vi "driveCode.vi"(6 "tankJoystick":enum16{"xbox", "twoJoystick"}(ring), 7 "mode":enum16{"Tank", "Split Arcade", "Arcade"}(ring)=enum."Arcade", 8 "driverJoystick2":T1={"Device"=enum."USB 1"}, 9 "driverJoystick1":T1={"Device"=enum."USB 1"}, 10 "rightDrive":T3={"DeviceStatus"={"status"=FALSE, "code"=0, "source"=""}, "Type"=enum."PWM", "PWM"={"PWM Channel"=enum."Invalid", "DeadBand"={"Name"="", "maxPositivePwm"=0, "minPositivePwm"=0, "centerPwm"=0, "maxNegativePwm"=0, "minNegativePwm"=0, "angularRange"=0}}, "CAN"={"Device Number"=0, "SetOutput VI Ref"=variant(refnum<vi> refnum), "GetOutput VI Ref"=variant(refnum<vi> refnum), "Enable VI Ref"=variant(refnum<vi> refnum), "Disable VI Ref"=variant(refnum<vi> refnum), "Data"=variant}, "Invert"=FALSE, "DIO PWM"={"PWM \"Enable\" Channel"=enum."Invalid", "DIOChannel"=enum."Invalid", "PWM Rate"=0.0}}, 11 "leftDrive":T3={"DeviceStatus"={"status"=FALSE, "code"=0, "source"=""}, "Type"=enum."PWM", "PWM"={"PWM Channel"=enum."Invalid", "DeadBand"={"Name"="", "maxPositivePwm"=0, "minPositivePwm"=0, "centerPwm"=0, "maxNegativePwm"=0, "minNegativePwm"=0, "angularRange"=0}}, "CAN"={"Device Number"=0, "SetOutput VI Ref"=variant(refnum<vi> refnum), "GetOutput VI Ref"=variant(refnum<vi> refnum), "Enable VI Ref"=variant(refnum<vi> refnum), "Disable VI Ref"=variant(refnum<vi> refnum), "Data"=variant}, "Invert"=FALSE, "DIO PWM"={"PWM \"Enable\" Channel"=enum."Invalid", "DIOChannel"=enum."Invalid", "PWM Rate"=0.0}}) -> (0 "rightSpeed (%)":dbl, 1 "rightDrive":T3={"DeviceStatus"={"status"=FALSE, "code"=0, "source"=""}, "Type"=enum."PWM", "PWM"={"PWM Channel"=enum."Invalid", "DeadBand"={"Name"="", "maxPositivePwm"=0, "minPositivePwm"=0, "centerPwm"=0, "maxNegativePwm"=0, "minNegativePwm"=0, "angularRange"=0}}, "CAN"={"Device Number"=0, "SetOutput VI Ref"=variant(refnum<vi> refnum), "GetOutput VI Ref"=variant(refnum<vi> refnum), "Enable VI Ref"=variant(refnum<vi> refnum), "Disable VI Ref"=variant(refnum<vi> refnum), "Data"=variant}, "Invert"=FALSE, "DIO PWM"={"PWM \"Enable\" Channel"=enum."Invalid", "DIOChannel"=enum."Invalid", "PWM Rate"=0.0}}, 2 "leftSpeed (%)":dbl, 3 "leftDrive":T3={"DeviceStatus"={"status"=FALSE, "code"=0, "source"=""}, "Type"=enum."PWM", "PWM"={"PWM Channel"=enum."Invalid", "DeadBand"={"Name"="", "maxPositivePwm"=0, "minPositivePwm"=0, "centerPwm"=0, "maxNegativePwm"=0, "minNegativePwm"=0, "angularRange"=0}}, "CAN"={"Device Number"=0, "SetOutput VI Ref"=variant(refnum<vi> refnum), "GetOutput VI Ref"=variant(refnum<vi> refnum), "Enable VI Ref"=variant(refnum<vi> refnum), "Disable VI Ref"=variant(refnum<vi> refnum), "Data"=variant}, "Invert"=FALSE, "DIO PWM"={"PWM \"Enable\" Channel"=enum."Invalid", "DIOChannel"=enum."Invalid", "PWM Rate"=0.0}})   [LabVIEW 2017]
uses:
  <vilib>/Rock Robotics/WPI/MotorControl/WPI_MotorControlDeviceRef.ctl
  <vilib>/Rock Robotics/WPI/MotorControl/WPI_MotorControlType.ctl
  <vilib>/Rock Robotics/SystemInterfaces/DIO/FPGA_DIOPWMChannel.ctl
  <vilib>/Rock Robotics/WPI/PWM/WPI_PWMDeadband.ctl
  <vilib>/Rock Robotics/SystemInterfaces/DIO/FPGA_DIOChannel.ctl
  <vilib>/Rock Robotics/WPI/Joystick/WPI_JoystickDevRef.ctl
  <vilib>/Rock Robotics/WPI/Joystick/WPI_JoystickDeviceEnum.ctl
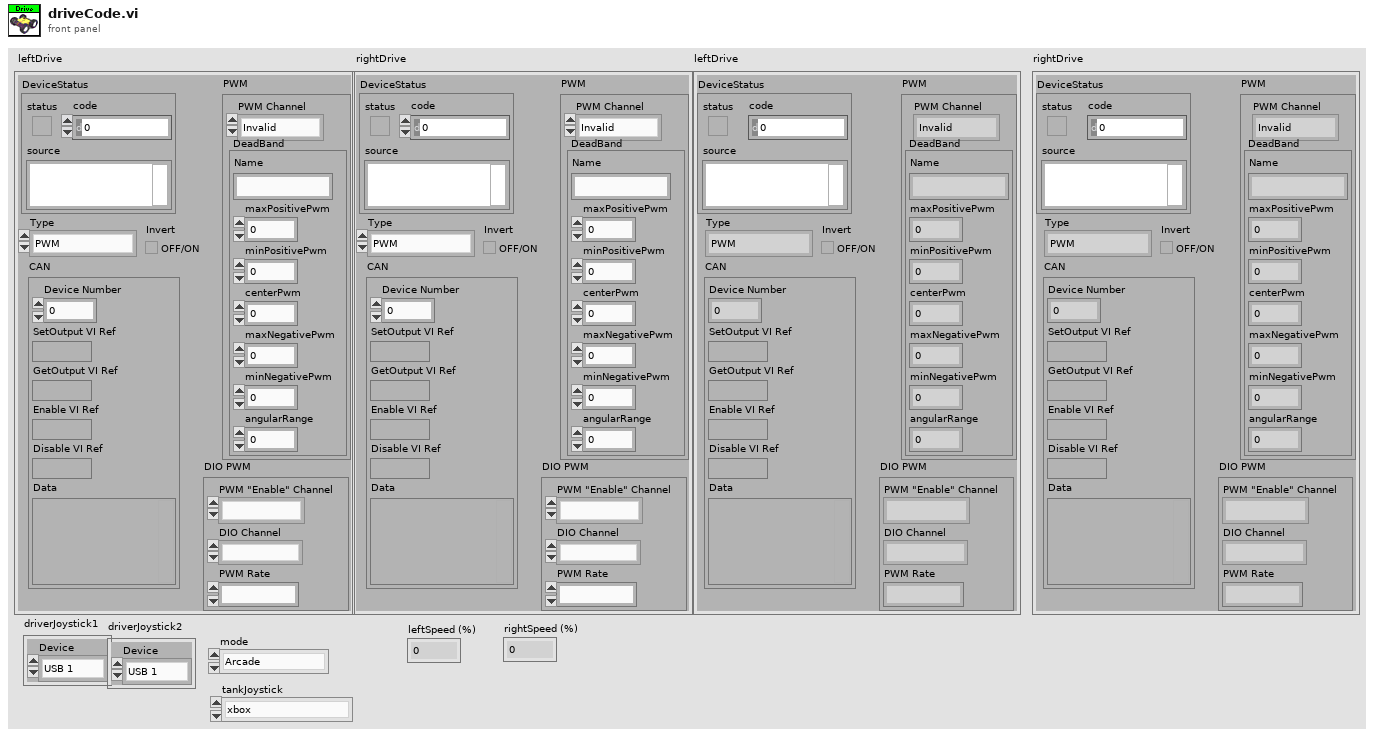
[diagram p1: front panel]
types:
  T1 = typedef "WPI_JoystickDevRef.ctl" = cluster{"Device":T2}
  T2 = typedef "WPI_JoystickDeviceEnum.ctl" = enum16{"USB 0", "USB 1", "USB 2", "USB 3", "USB 4", "USB 5"}
  T3 = typedef "WPI_MotorControlDeviceRef.ctl" = cluster{"DeviceStatus":errorcluster, "Type":T4, "PWM":cluster{"PWM Channel":T5, "DeadBand":T6}, "CAN":cluster{"Device Number":u8, "SetOutput VI Ref":variant, "GetOutput VI Ref":variant, "Enable VI Ref":variant, "Disable VI Ref":variant, "Data":variant}, "Invert":bool, "DIO PWM":cluster{"PWM \"Enable\" Channel":T5, "DIOChannel":T7, "PWM Rate":dbl}}
  T4 = typedef "WPI_MotorControlType.ctl" = enum16{"PWM", "CAN", "DIO PWM"}
  T5 = typedef "FPGA_DIOPWMChannel.ctl" = enum8{"PWM 0", "PWM 1", "PWM 2", "PWM 3", "PWM 4", "PWM 5", "PWM 6", "PWM 7", "PWM 8", "PWM 9", "PWM MXP 0", "PWM MXP 1", "PWM MXP 2", "PWM MXP 3", "PWM MXP 4", "PWM MXP 5", "PWM MXP 6", "PWM MXP 7", "PWM MXP 8", "PWM MXP 9", "Invalid"}
  T6 = typedef "WPI_PWMDeadband.ctl" = cluster{"Name":string, "maxPositivePwm":i32, "minPositivePwm":i32, "centerPwm":i32, "maxNegativePwm":i32, "minNegativePwm":i32, "angularRange":u16}
  T7 = typedef "FPGA_DIOChannel.ctl" = enum8{"DIO 0", "DIO 1", "DIO 2", "DIO 3", "DIO 4", "DIO 5", "DIO 6", "DIO 7", "DIO 8", "DIO 9", "DIO MXP 0", "DIO MXP 1", "DIO MXP 2", "DIO MXP 3", "DIO MXP 4", "DIO MXP 5", "DIO MXP 6", "DIO MXP 7", "DIO MXP 8", "DIO MXP 9", "DIO MXP 10", "DIO MXP 11", "DIO MXP 12", "DIO MXP 13", "DIO MXP 14", "DIO MXP 15", "SPI Port CS1", "SPI Port CS2", "SPI Port CS3", "SPI Port MISO", "SPI Port MOSI", "Invalid"}
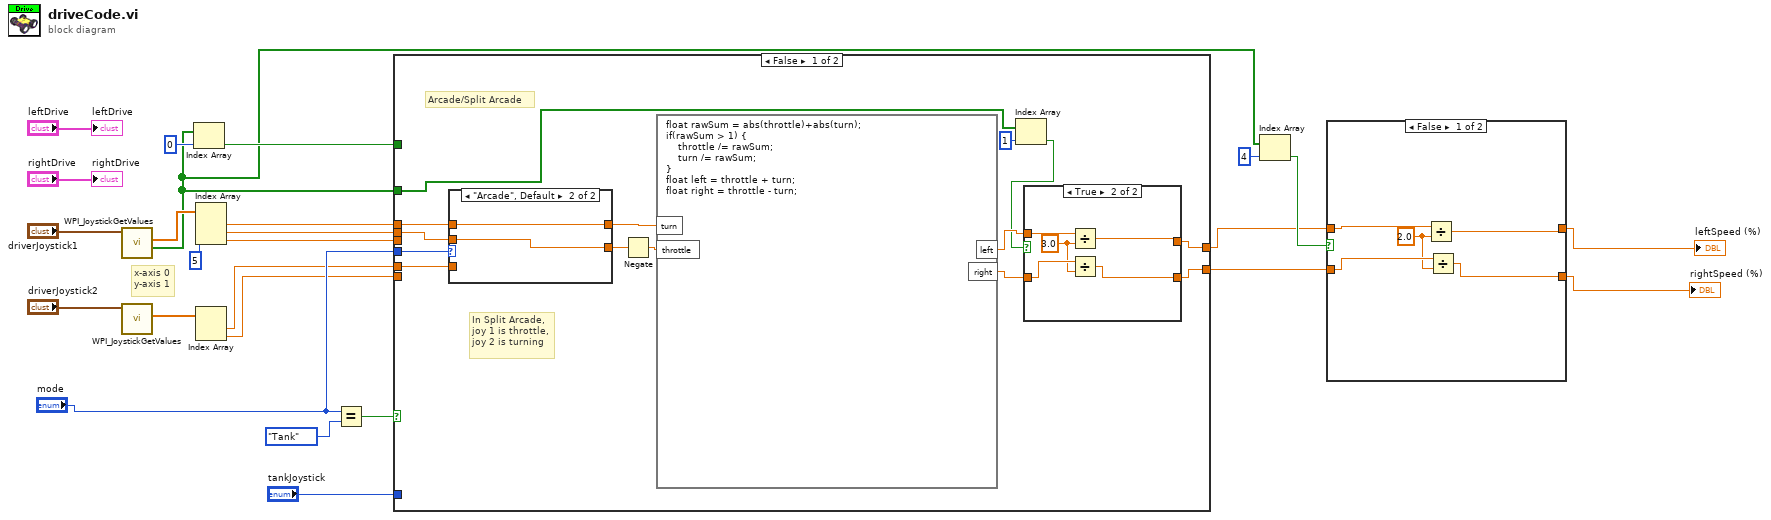
[diagram p0: block diagram]
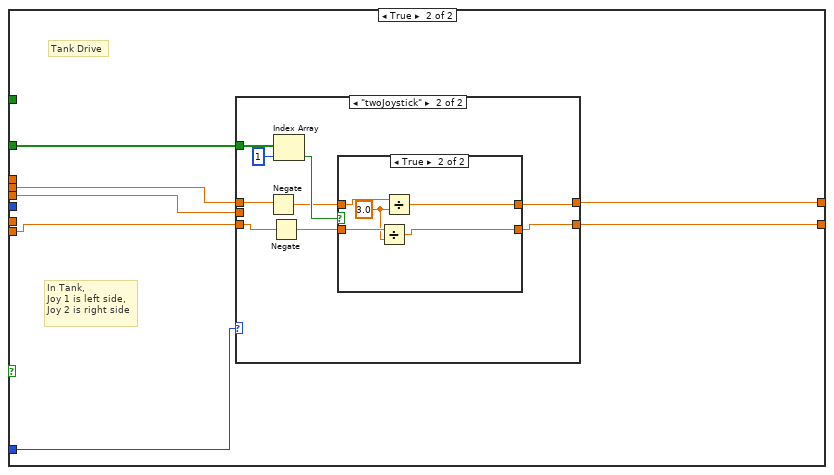
[diagram p5: hidden frame]
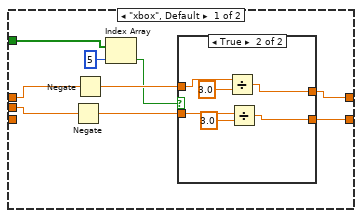
[diagram p6: hidden frame]
diagram:
  # "x-axis 0\ny-axis 1"
  n1 = call <vilib>:"WPI_JoystickGetValues.vi"("JoystickDevRef"="driverJoystick1") -> ("Buttons"=w7:bool[], "Axes"=w8:dbl[])  [unwired: 6 in, 3 out]
  n2 = call <vilib>:"WPI_JoystickGetValues.vi"("JoystickDevRef"="driverJoystick2") -> ("Axes"=w21:dbl[])  [unwired: 6 in, 4 out]
  n3 = Index Array(array=w7, index=0) -> (element=w13:bool)
  n4 = Index Array(array=w8, index #3=5 ("index")) -> (element #1=w17:dbl, element #2=w16:dbl, element #3=w9:dbl)  [unwired: 2 in]
  n5 = Index Array(array=w21) -> (element #1=w15:dbl, element #2=w14:dbl)  [unwired: 2 in]
  n6 = Equal?(x="mode", y=enum16{"Tank", "Split Arcade", "Arcade"}."Tank") -> (x = y?=w19:bool)
  n7 = case shown="False" w19 {
    tunnel: "mode" -> [w39 _]
    tunnel: w17 -> [w38 _]
    tunnel: w16 -> [w37 w56]
    tunnel: w15 -> [w35 _]
    tunnel: [w30 w55] -> w4
    tunnel: [w29 w54] -> w2
    tunnel: w14 -> [_ w57]
    tunnel: w13 -> [_ _]
    tunnel: "tankJoystick" -> [_ w53]
    tunnel: w9 -> [_ w52]
    tunnel: w7 -> [w28 w51]
    frame False {
      # "In Split Arcade,\njoy 1 is throttle,\njoy 2 is turning"
      # "Arcade/Split Arcade"
      n8 = case shown="\"Arcade\", Default" w39 {
        tunnel: w38 -> [_ w50]
        tunnel: w37 -> [w48 w49]
        tunnel: [w47 w50] -> w36
        tunnel: [w48 w49] -> w34
        tunnel: w35 -> [w47 _]
        frame "Split Arcade" {
        }
        frame "Arcade", Default {
        }
      }
      n9 = Negate(x=w34) -> (-x=w33:dbl)
      n10 = formula code="float rawSum = abs(throttle)+abs(turn);\nif(rawSum > 1) {\n    throttle /= rawSum;\n    turn /= rawSum;\n}\nfloat left = throttle + turn;\nfloat right = throttle - turn;"("turn"=w36, "throttle"=w33) -> ("left"=w32:dbl, "right"=w31:dbl)
      n11 = Index Array(array=w28, index=1) -> (element=w26:bool)
      n12 = case shown="True" w26 {
        tunnel: w32 -> [w41 w46]
        tunnel: w31 -> [w40 w45]
        tunnel: [w41 w43] -> w30
        tunnel: [w40 w42] -> w29
        frame False {
        }
        frame True {
          w44 = 3.0 ("y")
          n13 = Divide(x=w46, y=w44) -> (x/y=w43:dbl)
          n14 = Divide(x=w45, y=w44) -> (x/y=w42:dbl)
        }
      }
    }
    frame True {
      # "In Tank,\nJoy 1 is left side,\nJoy 2 is right side"
      # "Tank Drive"
      n15 = case shown="\"twoJoystick\"" w53 {
        tunnel: w57 -> [_ w75]
        tunnel: w56 -> [w66 w80]
        tunnel: [w62 w78] -> w55
        tunnel: [w61 w77] -> w54
        tunnel: w52 -> [w65 _]
        tunnel: w51 -> [w60 w83]
        frame "xbox", Default {
          n16 = Negate(x=w65) -> (-x=w63:dbl)
          n17 = Negate(x=w66) -> (-x=w64:dbl)
          n18 = Index Array(array=w60, index=5) -> (element=w58:bool)
          n19 = case shown="True" w58 {
            tunnel: w64 -> [w68 w74]
            tunnel: w63 -> [w67 w73]
            tunnel: [w68 w70] -> w62
            tunnel: [w67 w69] -> w61
            frame False {
            }
            frame True {
              n20 = Divide(x=w74, y=3.0) -> (x/y=w70:dbl)
              n21 = Divide(x=w73, y=3.0) -> (x/y=w69:dbl)
            }
          }
        }
        frame "twoJoystick" {
          n22 = Negate(x=w80) -> (-x=w79:dbl)
          n23 = Negate(x=w75) -> (-x=w76:dbl)
          n24 = Index Array(array=w83, index=1) -> (element=w81:bool)
          n25 = case shown="True" w81 {
            tunnel: w79 -> [w85 w90]
            tunnel: w76 -> [w84 w89]
            tunnel: [w85 w88] -> w78
            tunnel: [w84 w87] -> w77
            frame False {
            }
            frame True {
              w86 = 3.0 ("y")
              n26 = Divide(x=w89, y=w86) -> (x/y=w87:dbl)
              n27 = Divide(x=w90, y=w86) -> (x/y=w88:dbl)
            }
          }
        }
      }
    }
  }
  n28 = Index Array(array=w7, index=4) -> (element=w5:bool)
  n29 = case shown="False" w5 {
    tunnel: [w92 w97] -> w3
    tunnel: w4 -> [w95 w97]
    tunnel: [w91 w96] -> w1
    tunnel: w2 -> [w94 w96]
    frame False {
      w93 = 2.0 ("y")
      n30 = Divide(x=w95, y=w93) -> (x/y=w92:dbl)
      n31 = Divide(x=w94, y=w93) -> (x/y=w91:dbl)
    }
    frame True {
    }
  }
  "leftSpeed (%)" <- w3
  "rightSpeed (%)" <- w1
  "leftDrive" <- "leftDrive"
  "rightDrive" <- "rightDrive"
